vi "Adder.vi"(7 "x":dbl) -> (8 "sum":dbl)   [LabVIEW 2017]
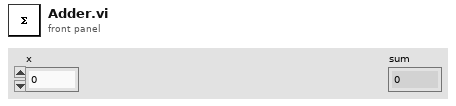
[diagram p1: front panel]
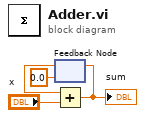
[diagram p0: block diagram]
diagram:
  n1 = feedback #1(0.0) -> (w3:dbl)
  n2 = Add(x=w3, y="x") -> (x+y=w4:dbl)
  "sum" <- w4
  n3 = feedback-in #1(w4) -> ()
